vi "Set Motor OFF ESP.vi"(8 "error in (no error)":errorcluster, 9 "Axis (1)":i32=1 min=1 max=3, 10 "VISA resource name":refnum<visa-resource-name>, 11 "ESP302 in":refnum<class "ESP302.lvclass">) -> (0 "error out":errorcluster, 2 "VISA resource name out":refnum<visa-resource-name>, 3 "ESP302 out":refnum<class "ESP302.lvclass">)   [LabVIEW 2020, in "ESP302.lvclass"]
uses:
  ESP302/ESP302.lvclass
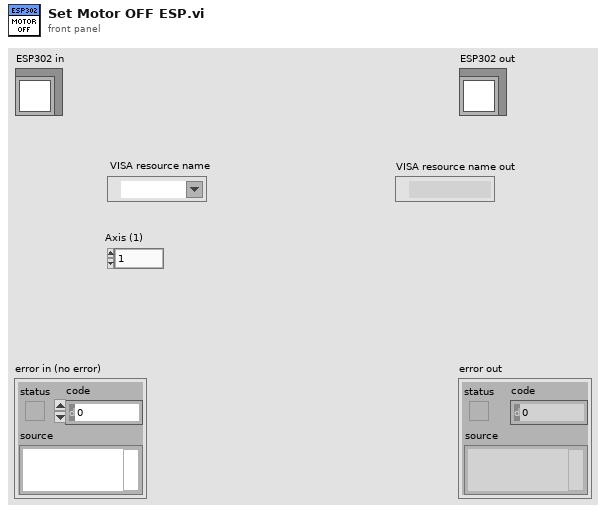
[diagram p1: front panel]
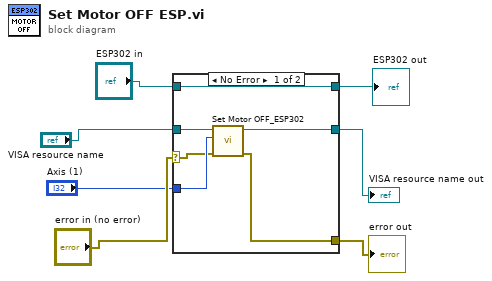
[diagram p0: block diagram]
diagram:
  n1 = case shown="No Error" "error in (no error)" {
    selector: "error in (no error)" -> [w10 w15]
    tunnel: "ESP302 in" -> [w13 w16]
    tunnel: [w13 w16] -> w6
    tunnel: [w9 w15] -> w5
    tunnel: "VISA resource name" -> [w12 w14]
    tunnel: "Axis (1)" -> [w11 _]
    tunnel: [w8 w14] -> w1
    frame No Error {
      n2 = call "Set Motor OFF_ESP302.vi"("error in (no error)"=w10, "Axis (1)"=w11, "VISA resource name"=w12) -> ("error out"=w9:errorcluster, "VISA resource name out"=w8:refnum<visa-resource-name>)  [unwired: 3 in]
    }
    frame Error {
    }
  }
  "error out" <- w5
  "ESP302 out" <- w6
  "VISA resource name out" <- w1
